vi "sub_cal_A5.vi"(11 "IR raw 2d":i16[][](array[numeric])) -> (3 "x+y":dbl[][](array[numeric]))   [LabVIEW 2013]
panel:
  out "x << y":u16[][](array[numeric])
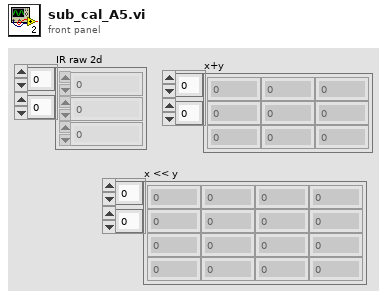
[diagram p1: front panel]
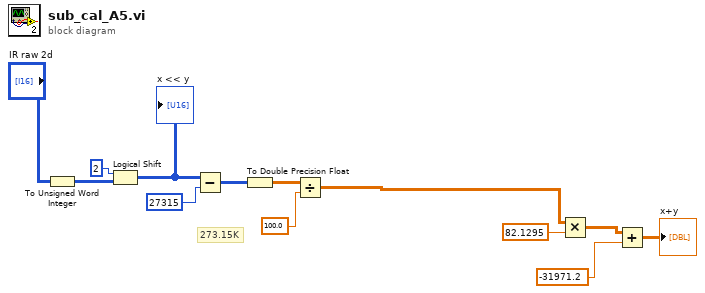
[diagram p0: block diagram]
diagram:
  # "273.15K"
  n1 = To Unsigned Word Integer(number="IR raw 2d") -> (unsigned 16bit integer=w9:u16[][])
  n2 = Logical Shift(y=i16 2, x=w9) -> (x << y=w2:u16[][])
  "x << y" <- w2
  n3 = Subtract(x=w2, y=u16 27315) -> (x-y=w11:u16[][])
  n4 = To Double Precision Float(number=w11) -> (double precision float=w1:dbl[][])
  n5 = Divide(x=w1, y=100.0) -> (x/y=w4:dbl[][])
  n6 = Multiply(x=w4, y=82.1295) -> (x*y=w7:dbl[][])
  n7 = Add(x=w7, y=-31971.2) -> (x+y=→"x+y":dbl[][])
